vi "Vision Processing.vi"(4 "error in (no error)":errorcluster, 7 "Image Size":T1=enum."320x240") -> ()   [LabVIEW 2013]
doc: "This VI runs in parallel to other tasks. It gets images from the camera, processes them for color or shape and use that information to affect robot behavior."
uses:
  <vilib>/Rock Robotics/WPI/Camera/WPI_CameraImageSize.ctl
  <vilib>/Rock Robotics/WPI/Camera/WPI_CameraWhite Balance Values.ctl
  <vilib>/Rock Robotics/WPI/Camera/WPI_CameraExposure Values.ctl
  <vilib>/Rock Robotics/WPI/Camera/WPI_CameraFrameRate.ctl
  Robot Global Data.vi
panel:
  in  "Reliable?":bool=TRUE
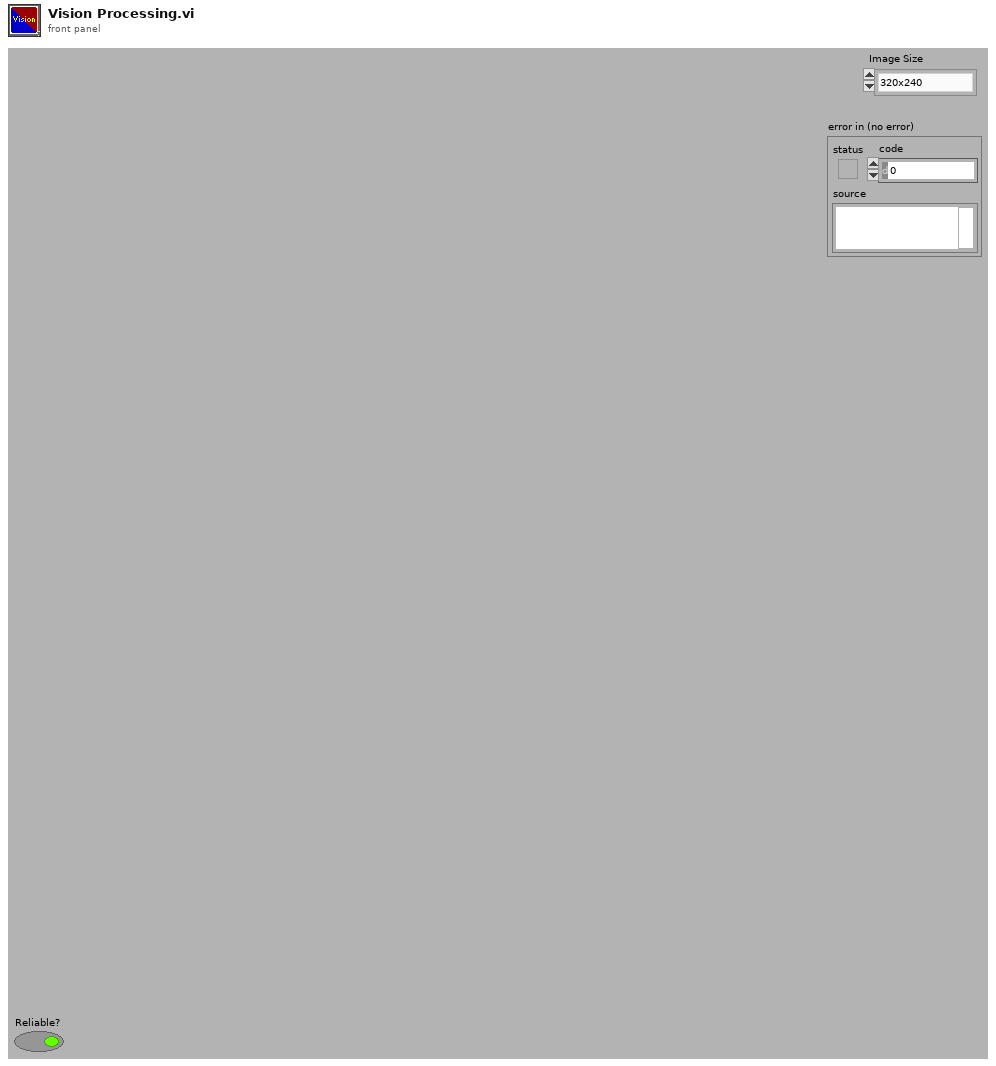
[diagram p1: front panel]
types:
  T1 = typedef "WPI_CameraImageSize.ctl" = enum16{"640x480", "320x240", "160x120"}
  T2 = typedef "WPI_CameraFrameRate.ctl" = u32
  T3 = typedef "WPI_CameraExposure Values.ctl" = enum16{"Auto", "Flicker-free 50 Hz", "Flicker-free 60 Hz", "Hold current"}
  T4 = typedef "WPI_CameraWhite Balance Values.ctl" = enum16{"Auto", "Fixed indoor", "Fixed outdoor 1", "Fixed outdoor 2", "Fixed fluorescent 1", "Fixed fluorescent 2", "Hold current"}
  T5 = typedef "Image Type" = u32
  T6 = typedef "WPI_CameraDevRef.ctl" = cluster{"Camera Address":string, "CameraStatus":errorcluster, "Acquire Image Notifier":refnum<notifier>}
  T7 = typedef "IMAQ Image.ctl" = refnum<image>
  T8 = typedef "WPI_DriverStationMatch Info.ctl" = cluster{"Autonomous Elapsed Seconds":dbl, "TeleOp Elapsed Seconds":dbl, "Disabled Elapsed Seconds":dbl, "Visited Autonomous":bool, "Visited TeleOp":bool, "Visited Disabled":bool, "Autonomous Settings":cluster{"Autonomous Style":enum16{"Iterative", "Independent"}, "VI Refnum":refnum<vi>}}
  T9 = typedef "WPI_DriverStationRobotMode2.ctl" = enum16{"Autonomous Disabled", "Autonomous Enabled", "Teleop Disabled", "Teleop Enabled", "Timeout", "Finish", "Test Disabled", "Test Enabled"}
  T10 = cluster{cluster{"Numeric":dbl, "Numeric":dbl}, cluster{"Numeric":dbl, "Numeric":dbl}, cluster{"Numeric":dbl, "Numeric":dbl}}
  T11 = cluster{"Horizontal":bool, "Aspect Score":dbl, "Rect Score":dbl, cluster{"Left":dbl, "Top":dbl, "Right":dbl, "Bottom":dbl}, "Equiv H":dbl, "Equiv V":dbl}[]
  T12 = typedef "TargetType.ctl" = enum16{"Not Hot", "Hot"}
  T13 = cluster{"Scores":cluster{"Total":dbl, "Left":dbl, "Right":dbl, "Ratio":dbl, "Vertical":dbl, "index":i32, "State":T12}, "Verticals":cluster{"Horizontal?":bool, "Aspect Score":dbl, "Rect Score":dbl, cluster{"Left":dbl, "Top":dbl, "Right":dbl, "Bottom":dbl}, "Equiv H":dbl, "Equiv V":dbl}, "Horizontals":cluster{"Horizontal?":bool, "Aspect Score":dbl, "Rect Score":dbl, cluster{"Left":dbl, "Top":dbl, "Right":dbl, "Bottom":dbl}, "Equiv H":dbl, "Equiv V":dbl}, "Validated":bool}[]
  T14 = cluster{"Scores":cluster{"Total":dbl, "Left":dbl, "Right":dbl, "Ratio":dbl, "Vertical":dbl, "index":i32, "State":T12}, "Verticals":cluster{"Horizontal?":bool, "Aspect Score":dbl, "Rect Score":dbl, cluster{"Left":dbl, "Top":dbl, "Right":dbl, "Bottom":dbl}, "Equiv H":dbl, "Equiv V":dbl}, "Horizontals":cluster{"Horizontal?":bool, "Aspect Score":dbl, "Rect Score":dbl, cluster{"Left":dbl, "Top":dbl, "Right":dbl, "Bottom":dbl}, "Equiv H":dbl, "Equiv V":dbl}, "Distance (ft)":dbl, "Target Center (-1 to 1)":cluster{"X":dbl, "Y":dbl}}[]
  T15 = cluster{"Scores":cluster{"Total":dbl, "Left":dbl, "Right":dbl, "Ratio":dbl, "Vertical":dbl, "index":i32, "State":T12}, "Verticals":cluster{"Horizontal?":bool, "Aspect Score":dbl, "Rect Score":dbl, cluster{"Left":dbl, "Top":dbl, "Right":dbl, "Bottom":dbl}, "Equiv H":dbl, "Equiv V":dbl}, "Horizontals":cluster{"Horizontal?":bool, "Aspect Score":dbl, "Rect Score":dbl, cluster{"Left":dbl, "Top":dbl, "Right":dbl, "Bottom":dbl}, "Equiv H":dbl, "Equiv V":dbl}, "Distance (ft)":dbl, "Target Center (-1 to 1)":cluster{"X":dbl, "Y":dbl}}
  T16 = cluster{"Total":dbl, "Left":dbl, "Right":dbl, "Ratio":dbl, "Vertical":dbl, "index":i32, "State":T12}
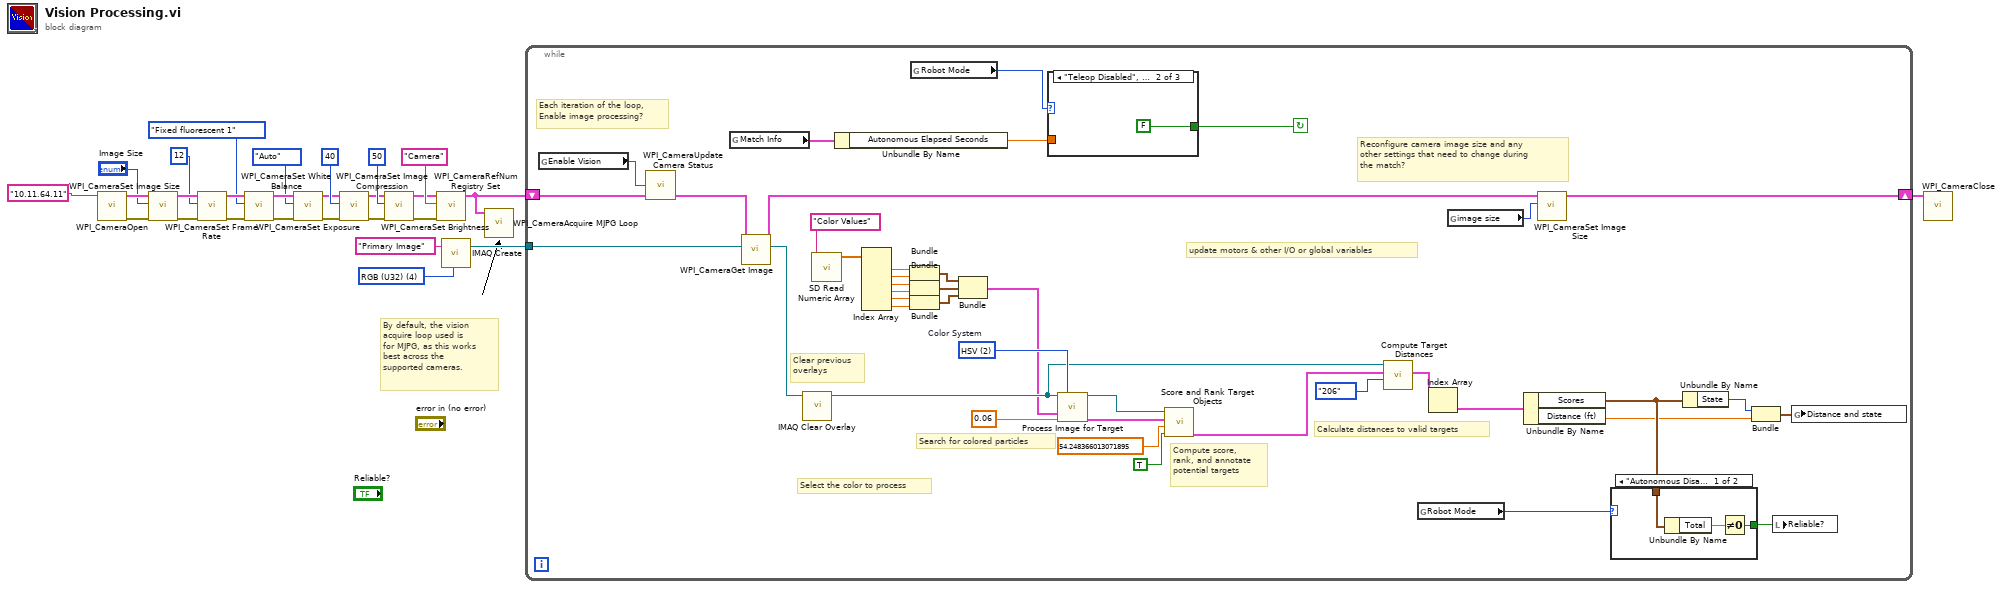
[diagram p0: block diagram]
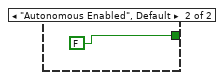
[diagram p2: hidden frame]
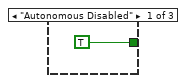
[diagram p3: hidden frame]
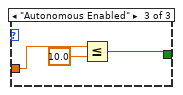
[diagram p4: hidden frame]
diagram:
  w27 = T5 4 items=["Grayscale (U8)", "Grayscale (I16)", "Grayscale (SGL)", "Complex (CSG)", "RGB (U32)", "HSL (U32)", "RGB (U64)"] ("Image Type")
  # "By default, the vision\nacquire loop used is\nfor MJPG, as this works\nbest across the\nsupported cameras."
  n1 = call <vilib>:"WPI_CameraOpen.vi"("Camera Address"="10.11.64.11" ("format string")) -> ("error out"=w15:errorcluster, "CameraDevRef"=w16:T6)  [unwired: 1 in, 8 out]
  n2 = call <vilib>:"WPI_CameraSet Image Size.vi"("error in (no error)"=w15, "Image Size"="Image Size", "CameraDevRef"=w16) -> ("error out"=w14:errorcluster, "CameraDevRef Out"=w17:T6)  [unwired: 7 out]
  n3 = call <vilib>:"WPI_CameraSet Frame Rate.vi"("error in (no error)"=w14, "Frame Rate (fps)"=T2 12, "CameraDevRef"=w17) -> ("error out"=w13:errorcluster, "CameraDevRef Out"=w19:T6)  [unwired: 7 out]
  n4 = call <vilib>:"WPI_CameraSet White Balance.vi"("error in (no error)"=w13, "White Balance"=WPI_CameraWhite_Balance_Values."Fixed fluorescent 1", "CameraDevRef"=w19) -> ("error out"=w12:errorcluster, "CameraDevRef Out"=w18:T6)  [unwired: 7 out]
  n5 = call <vilib>:"WPI_CameraSet Exposure.vi"("error in (no error)"=w12, "Exposure"=WPI_CameraExposure_Values."Auto", "CameraDevRef"=w18) -> ("error out"=w11:errorcluster, "CameraDevRef Out"=w21:T6)  [unwired: 7 out]
  n6 = call <vilib>:"WPI_CameraSet Image Compression.vi"("error in (no error)"=w11, "Compression"=40, "CameraDevRef"=w21) -> ("error out"=w10:errorcluster, "CameraDevRef Out"=w20:T6)  [unwired: 7 out]
  n7 = call <vilib>:"WPI_CameraSet Brightness.vi"("error in (no error)"=w10, "Brightness"=50, "CameraDevRef"=w20) -> ("error out"=w8:errorcluster, "CameraDevRef Out"=w9:T6)  [unwired: 7 out]
  n8 = call <vilib>:"WPI_CameraRefNum Registry Set.vi"("error in (no error)"=w8, "refnum name"="Camera", "CameraDevRef"=w9) -> ("CameraDevRef"=w4:T6)  [unwired: 8 out]
  n9 = call "IMAQ Create"("Image Name"="Primary Image", "Image Type"=w27) -> ("New Image"=w25:T7)  [unwired: 2 in, 2 out]
  n10 = call <vilib>:"WPI_CameraAcquire MJPG Loop.vi"("CameraDevRef"=w4) -> ()  [unwired: 11 in]
  n11 = while {
    tunnel: w25 -> [w68]
    shift-right: [w47] -> w1
    shift-left: w4 -> [w67]
    stop <- w49 continue-if-true
    w56 = u16 2 items=["RGB", "HSL", "HSV", "HSI"]  # Color System
    # "Clear previous\noverlays"
    # "Calculate distances to valid targets"
    # "Search for colored particles"
    # "Compute score,\nrank, and annotate\npotential targets"
    # "Select the color to process"
    # "update motors & other I/O or global variables"
    # "Reconfigure camera image size and any\nother settings that need to change during\nthe match?"
    # "Each iteration of the loop,\nEnable image processing?"
    n12 = global read "Robot Global Data.vi" "Enable Vision"() -> (w65:bool)
    n13 = call <vilib>:"WPI_CameraUpdate Camera Status.vi"("CameraDevRef In"=w67, "Enable Vision"=w65) -> ("CameraDevRef Out"=w66:T6)  [unwired: 3 in]
    n14 = global read "Robot Global Data.vi" "Match Info"() -> (w44:T8)
    n15 = call <vilib>:"WPI_CameraGet Image.vi"("Image"=w68, "CameraDevRef"=w66) -> ("Image Out"=w53:T7, "CameraDevRef Out"=w63:T6)  [unwired: 1 in, 7 out]
    n16 = call "IMAQ Clear Overlay"("Image"=w53) -> ("Image Out"=w55:T7)  [unwired: 9 in, 1 out]
    n17 = call <vilib>:"SD Read Numeric Array.vi"("Name"="Color Values") -> ("Numeric Array"=w43:dbl[])  [unwired: 8 in, 2 out]
    n18 = Unbundle By Name(w44) -> ("Autonomous Elapsed Seconds"=w48:dbl)
    n19 = Index Array(array=w43) -> (element #1=w41:dbl, element #2=w42:dbl, element #3=w40:dbl, element #4=w39:dbl, element #5=w38:dbl, element #6=w37:dbl)  [unwired: 6 in]
    n20 = Bundle("Numeric"=w41, "Numeric"=w42) -> (w36:cluster{"Numeric":dbl, "Numeric":dbl})  [unwired: 1 in]
    n21 = Bundle("Numeric"=w40, "Numeric"=w39) -> (w35:cluster{"Numeric":dbl, "Numeric":dbl})  [unwired: 1 in]
    n22 = Bundle("Numeric"=w38, "Numeric"=w37) -> (w34:cluster{"Numeric":dbl, "Numeric":dbl})  [unwired: 1 in]
    n23 = global read "Robot Global Data.vi" "Robot Mode"() -> (w50:T9)
    n24 = Bundle(w36, w35, w34) -> (w33:T10)  [unwired: 1 in]
    n25 = case shown="\"Teleop Disabled\", Default" w50 {
      tunnel: [TRUE FALSE w77] -> w49
      tunnel: w48 -> [_ _ w75]
      frame "Autonomous Disabled" {
      }
      frame "Teleop Disabled", Default {
      }
      frame "Autonomous Enabled" {
        n26 = Less Or Equal?(x=w75, y=10.0) -> (x <= y?=w77:bool)
      }
    }
    n27 = call "Process Image for Target.vi"("Src Image"=w55, "Color Mode"=w56, "Color Components"=w33, "Area Cutoff %"=0.06 ("Area Size Limit %")) -> ("Src Image Out"=w61:T7, "Particles"=w59:T11)  [unwired: 6 in, 4 out]
    n28 = call "Score and Rank Target Objects.vi"("Annotate"=TRUE, "Score Limit"=54.248366013071895 ("Score Cutoff"), "Particles"=w59, "Image in"=w61) -> ("Target Info"=w58:T13)  [unwired: 6 in, 1 out]
    n29 = call "Compute Target Distances.vi"("Camera Type"=enum16{"206", "1011", "1013"}."206", "Target Info"=w58, "Image in"=w55) -> ("Target Info"=w52:T14)  [unwired: 6 in, 2 out]
    n30 = global read "Robot Global Data.vi" "Robot Mode"() -> (w46:T9)
    n31 = Index Array(array=w52) -> (element=w51:T15)  [unwired: 1 in]
    n32 = global read "Robot Global Data.vi" "image size"() -> (w64:T1)
    n33 = Unbundle By Name(w51) -> ("Scores"=w45:T16, "Distance (ft)"=w29:dbl)
    n34 = call <vilib>:"WPI_CameraSet Image Size.vi"("Image Size"=w64, "CameraDevRef"=w63) -> ("CameraDevRef Out"=w47:T6)  [unwired: 1 in, 8 out]
    n35 = case shown="\"Autonomous Disabled\"" w46 {
      tunnel: w45 -> [w71 _]
      tunnel: [w69 FALSE ("Reliable? 2")] -> w31
      frame "Autonomous Disabled" {
        n36 = Unbundle By Name(w71) -> ("Total"=w70:dbl)
        n37 = Not Equal To 0?(x=w70) -> (x != 0?=w69:bool)
      }
      frame "Autonomous Enabled", Default {
      }
    }
    n38 = Unbundle By Name(w45) -> ("State"=w30:T12)
    n39 = Bundle("State"=w30, "Distance (ft)"=w29) -> (w28:cluster{"State":T12, "Distance (ft)":dbl})  [unwired: 1 in]
    n40 = local write "Reliable?"(w31) -> ()
    n41 = global write "Robot Global Data.vi" "Distance and state"(w28) -> ()
  }
  n42 = call <vilib>:"WPI_CameraClose.vi"("CameraDevRef"=w1) -> ()  [unwired: 1 in, 10 out]
